vi "control_PI.vi"() -> ()   [LabVIEW 2022 SP3]
uses:
  <vilib>/Utility/NIReport.llb/Report Type.ctl
  <vilib>/imath/engines/lvmath/Plug In/_Char/NIMS_CH_character datatype.ctl
  <vilib>/imath/engines/lvmath2/RunTimeEngine/Managers/WorkSpace/UID Generator.vi
  <vilib>/imath/engines/lvmath2/RunTimeEngine/RunTimeType/NIMS_RunTimeType_From StrictType (excl LVString).vi
  <instcachedir>/0/NIMS_RunTimeType_From StrictType (excl LVString)_70DEE8F51B6B495C85F505DE4E7061F1.lvgen/NIMS_RunTimeType_From StrictType (excl LVString)_70DEE8F51B6B495C85F505DE4E7061F1_000.vi
  <vilib>/imath/engines/lvmath2/RunTimeEngine/LocalVariableDefStatement/MC_LocalVariableDefStatement_Display.vi
  <vilib>/imath/engines/lvmath/Plug In/_Char/NIMS_CH_Character 1D to U8 1D.vi
  <vilib>/imath/engines/lvmath/Plug In/Control Design/BuiltInFunctions/tf/NIMS_CD_tf({num},{den}).vi
  <instcachedir>/0/NIMS_CD_tf({num},{den})_2A4567CC0C2B4A37A239C252B1516632.lvgen/NIMS_CD_tf({num},{den})_2A4567CC0C2B4A37A239C252B1516632_000.vi
  <instcachedir>/0/NIMS_RunTimeType_From StrictType (excl LVString)_70DEE8F51B6B495C85F505DE4E7061F1.lvgen/NIMS_RunTimeType_From StrictType (excl LVString)_70DEE8F51B6B495C85F505DE4E7061F1_031.vi
  <vilib>/imath/engines/lvmath2/RunTimeEngine/IndexRead/NIMS V(S).vi
  <instcachedir>/0/NIMS V(S)_0488751826AF41519A22953C041130DC.lvgen/NIMS V(S)_0488751826AF41519A22953C041130DC_000.vi
  <vilib>/imathl/engines/lvmath/Functions/Error Handling/Create Error.vi
  <vilib>/imath/engines/lvmath2/RunTimeEngine/Managers/SymbolTable/Clear UID.vi
  <vilib>/imath/engines/lvmath2/RunTimeEngine/NodeEndStatement/NIMS_NodeEndStatement_Output.vi
  <instcachedir>/0/NIMS_NodeEndStatement_Output_53EC0D466D134D7ABD903AC30B43404B.lvgen/NIMS_NodeEndStatement_Output_53EC0D466D134D7ABD903AC30B43404B_001.vi
  <vilib>/imath/engines/lvmath2/RunTimeEngine/ErrorHandling/NIMS_Finalize Error.vi
  <vilib>/addons/_office/excel.llb/Excel Easy Table (num).vi
  <vilib>/Utility/NIReport.llb/NI_report.lvclass
  <vilib>/imath/engines/lvmath2/RunTimeEngine/Managers/SymbolTable/NIMS_WorkSpace.lvlib
  <vilib>/Utility/NIReport.llb/NI_ReportGenerationCore.lvlib
  <vilib>/addons/_office/NI_ReportGenerationToolkit.lvlib
  <vilib>/Utility/NIReport.llb/Excel/NI_Excel.lvclass
panel:
  out "Error":dbl
  out "AC":dbl
  out "SP":dbl
  out "q2":dbl
  out "q1":dbl
  out "q0":dbl
  in  "Perturbacion":bool
  in  "?":path
  in  "?":bool
  out "Temperature":dbl
  out "?":cluster{"y_k":dbl, "Int r":dbl, "uk":dbl, dbl}(graph)
  in  "SP":dbl
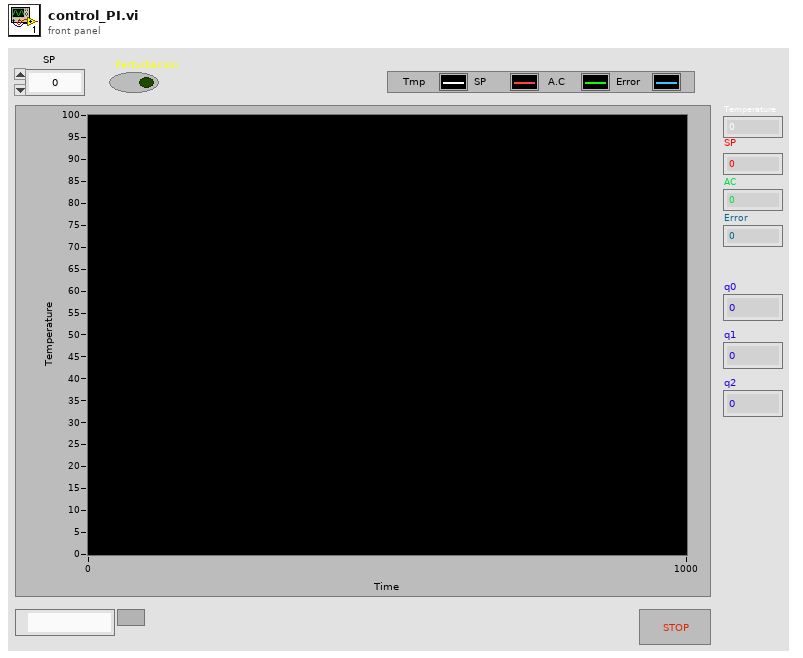
[diagram p1: front panel]
types:
  T1 = typedef "NI_ReportGenerationCore.lvlib/Report Type.ctl" = enum16{"HTML", "Word", "Excel"}
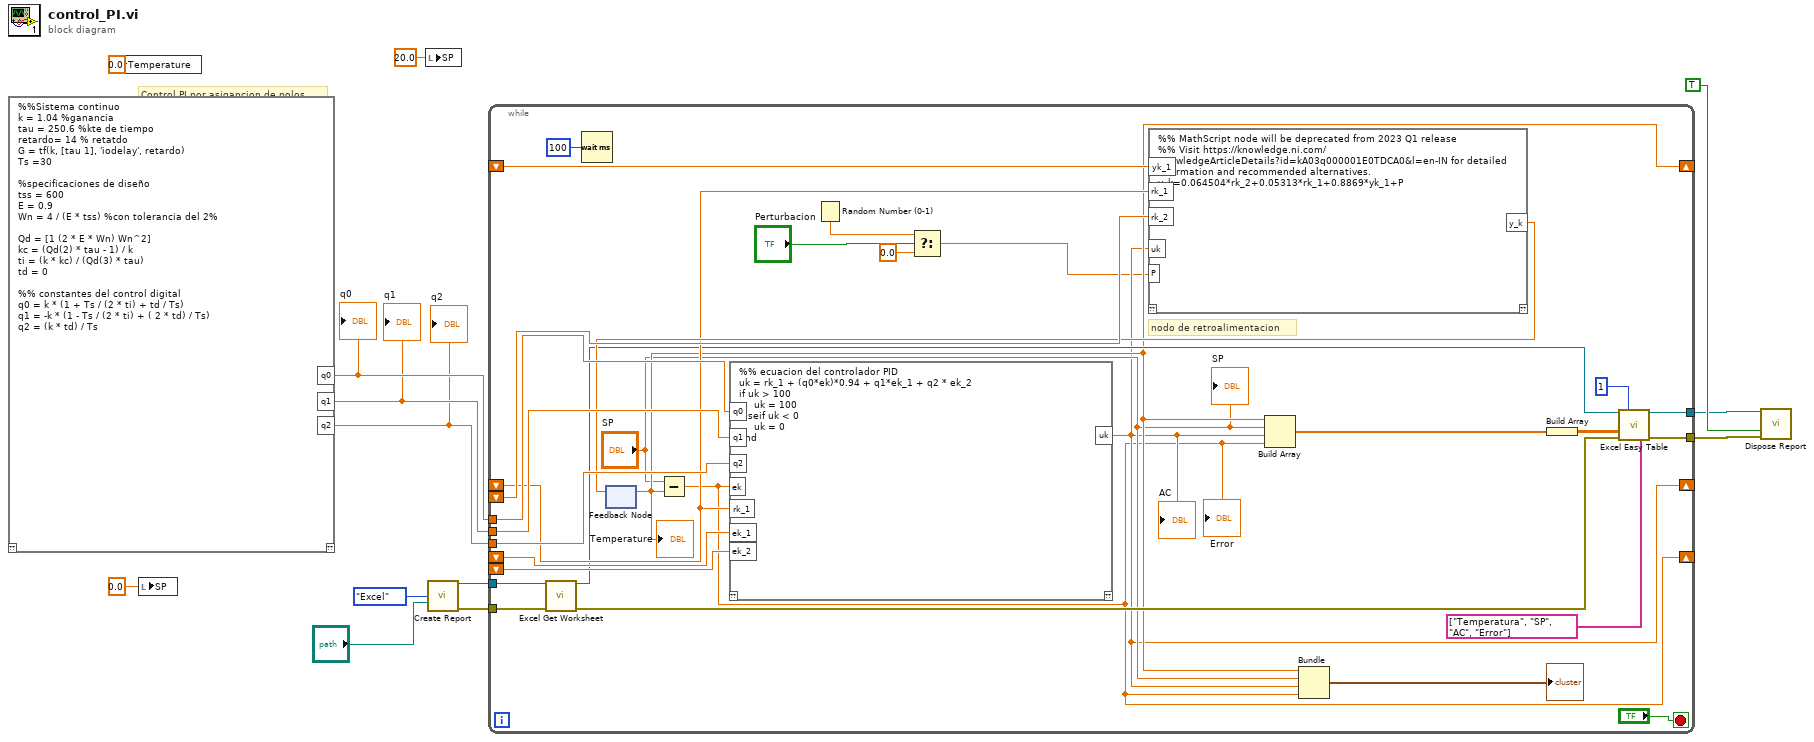
[diagram p0: block diagram]
diagram:
  # "Control PI por asigancion de polos"
  n1 = mathscript code="%%Sistema continuo\nk = 1.04 %ganancia\ntau = 250.6 %kte de tiempo\nretardo= 14 % retatdo\nG = tf(k, [tau 1], 'iodelay', retardo)\nTs =30\n\n%specificaciones de diseño\ntss = 600\nE = 0.9\nWn = 4 / (E * tss) %con tolerancia del 2%\n\nQd = [1 (2 * E * Wn) Wn^2]\nkc = (Qd(2) * tau - 1) / k\nti = (k * kc) / (Qd(3) * tau)\ntd = 0\n\n%% constantes del control digital\nq0 = k * (1 + Ts / (2 * ti) + td / Ts)\nq1 = -k * (1 - Ts / (2 * ti) + ( 2 * td) / Ts)\nq2 = (k * td) / Ts"() -> ("q0"=w11:dbl, "q1"=w10:dbl, "q2"=w9:dbl)  [unwired: 1 in, 1 out]
  "q0" <- w11
  "q1" <- w10
  "q2" <- w9
  n2 = local write "Temperature"(0.0 ("y_k")) -> ()
  n3 = local write "SP"(0.0 ("Int r")) -> ()
  n4 = local write "SP"(20.0 ("SP")) -> ()
  n5 = call <vilib>:"Create Report.vi"("report type"=Report_Type."Excel", "template (empty)"="?") -> ("report out"=w5:refnum<class "NI_report.lvclass">, "error out"=w4:errorcluster)  [unwired: 12 in]
  n6 = while {
    shift-right: [w23] -> _
    shift-left: _ -> [w36]
    shift-right: [w21] -> _
    shift-left: _ -> [w35]
    shift-left: _ -> [w43]
    tunnel: w11 -> [w40]
    tunnel: w10 -> [w39]
    tunnel: w9 -> [w38]
    shift-right: [w20] -> _
    shift-left: _ -> [w34]
    shift-left: _ -> [w33]
    tunnel: w5 -> [w27]
    tunnel: w4 -> [w26]
    tunnel: [w25] -> w3
    tunnel: [w24] -> w2
    stop <- "?" stop-if-true
    # "nodo de retroalimentacion"
    n7 = call <vilib>:"Excel Get Worksheet.vi"("report in"=w27, "error in (no error)"=w26) -> ("report out"=w30:refnum<class "NI_report.lvclass">, "error out"=w31:errorcluster)  [unwired: 12 in]
    n8 = Wait (ms)(milliseconds to wait=u32 100) -> ()  [unwired: 1 out]
    n9 = feedback #1() -> (w23:dbl)  [unwired: 1 in]
    "Temperature" <- w23
    n10 = Subtract(x="SP", y=w23) -> (x-y=w20:dbl)
    "Error" <- w20
    n11 = mathscript code="%% ecuacion del controlador PID\nuk = rk_1 + (q0*ek)*0.94 + q1*ek_1 + q2 * ek_2\nif uk > 100\n     uk = 100\nelseif uk < 0\n     uk = 0 \nend"("q0"=w40, "q1"=w39, "q2"=w38, "ek"=w20, "rk_1"=w35, "ek_1"=w34, "ek_2"=w33) -> ("uk"=w21:dbl)  [unwired: 1 in, 1 out]
    "AC" <- w21
    n12 = Random Number (0-1)() -> (number: 0 to 1=w17:dbl)
    n13 = Select(t=w17, s="Perturbacion", f=0.0) -> (s? t:f=w14:dbl)
    n14 = mathscript code="%% MathScript node will be deprecated from 2023 Q1 release\n%% Visit https://knowledge.ni.com/KnowledgeArticleDetails?id=kA03q000001E0TDCA0&l=en-IN for detailed information and recommended alternatives.\ny_k=0.064504*rk_2+0.05313*rk_1+0.8869*yk_1+P"("yk_1"=w36, "rk_1"=w35, "rk_2"=w43, "uk"=w21, "P"=w14) -> ("y_k"=w37:dbl)  [unwired: 1 in, 1 out]
    n15 = feedback-in #1(w37) -> ()
    n16 = Build Array(w23, "SP", w21, w20) -> (w19:dbl[])
    n17 = Bundle("y_k"=w23, "SP"="SP", "uk"=w21, w20) -> (→"?":cluster{"y_k":dbl, "SP ":dbl, "uk":dbl, dbl})  [unwired: 1 in]
    n18 = Build Array(w19) -> (w18:dbl[][])
    n19 = call-poly <vilib>:"Excel Easy Table.vi"("report in"=w30, "iteration"=1, "text data"=w18, "error in (no error)"=w31, "column headers"=string[] ["Temperatura", "SP", "AC", "Error"]) -> ("report out"=w25:refnum<class "NI_report.lvclass">, "error out"=w24:errorcluster)  [unwired: 6 in, 3 out]
    "SP" <- "SP"
  }
  n20 = call-dynamic "Dispose Report.vi"("report in"=w3, "save changes? (F)"=TRUE, "error in (no error)"=w2) -> ()  [unwired: 12 in, 1 out]
